vi "OAT Polar PG angle lines.vi"(6 "channel settings":T1 {"probe angle [deg]" max=360 step=1; "shaft rotating direction" items=["CCW", "CW"]}, 8 "grid measurements":T2 {"end angle" format="%.2f"; "start angle" format="%.2f"; "scale factors"."b" format="%.2f"; "scale factors"."a" format="%.2f"}, 9 "decade specs":cluster{"radius":i16, "label":string}[](array[cluster]), 11 "picture":picture) -> (3 "new picture":picture)   [LabVIEW 2017]
panel:
  in  "?":cluster{"angle":dbl, "min radius":i16}[](array[cluster])=[{"angle"=0.0, "min radius"=0}, {"angle"=15.0, "min radius"=25}, {"angle"=30.0, "min radius"=25}, {"angle"=45.0, "min radius"=10}, {"angle"=60.0, "min radius"=25}, {"angle"=75.0, "min radius"=25}] {"angle" format="%.2f"}
  # "To change the number of\nangle lines drawn add or\nremove elements from\nthis array.  (Changes\nwill only be temporary\nunless you make the new\nvalue the default and save\nthe VI.)\n\nAngle refers to the angle\nof the line in degrees.  The\nangles should be >=0 and\n<90, as these values are\nrepeated for each quadrant.\n\nMin radius refers to the\nsmallest size circle the\nlines should be drawn to."
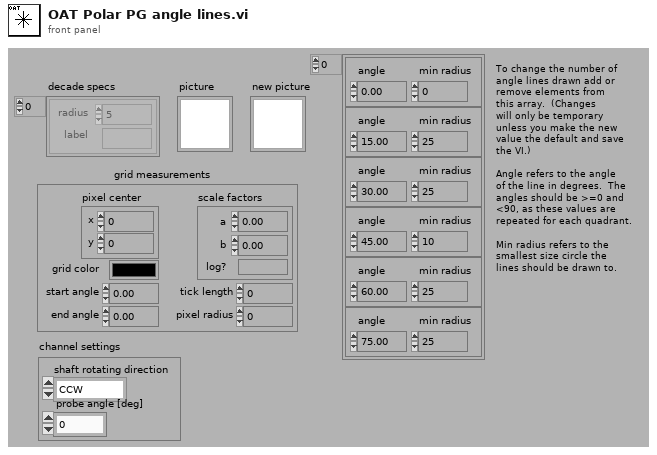
[diagram p1: front panel]
types:
  T1 = cluster{"shaft rotating direction":u16, "probe angle [deg]":u16}
  T2 = cluster{"pixel center":cluster{"x":i16, "y":i16}, "scale factors":cluster{"a":dbl, "b":dbl, "log?":bool}, "grid color":u32, "start angle":dbl, "end angle":dbl, "tick length":i16, "pixel radius":i32}
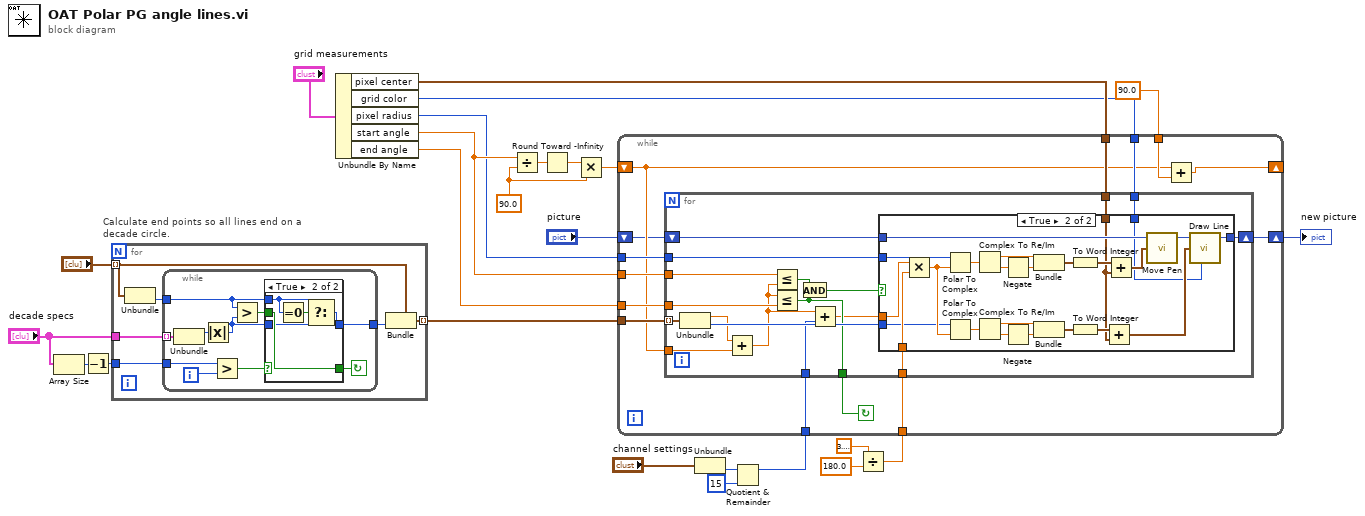
[diagram p0: block diagram]
diagram:
  w5 = 90.0
  n1 = Array Size(array="decade specs") -> (size(s)=w22:i32)
  n2 = Decrement(x=w22) -> (x-1=w20:i32)
  n3 = for "Calculate end points so all lines end on a decade circle." {
    tunnel: "?" -> [w28] mode=indexing
    tunnel: "decade specs" -> [w31]
    tunnel: w20 -> [w30]
    tunnel: [w26] -> w10 mode=indexing
    n4 = Unbundle(w28) -> ("min radius"=w29:i16)  [unwired: 1 out]
    n5 = while {
      tunnel: [w34] -> w27
      tunnel: w29 -> [w33]
      tunnel: w30 -> [w39]
      tunnel: w31 -> [w41] mode=indexing
      i -> [w40]
      stop <- w37 continue-if-true
      n6 = Unbundle(w41) -> ("radius"=w36:i16)  [unwired: 1 out]
      n7 = Absolute Value(x=w36) -> (abs(x)=w32:i16)
      n8 = Greater?(x=w39, y=w40) -> (0:w38:bool)
      n9 = Greater?(x=w33, y=w32) -> (0:w35:bool)
      n10 = case shown="True" w38 {
        selector: w38 -> [w43 _]
        tunnel: [w43 w48] -> w37
        tunnel: w32 -> [w42 w44]
        tunnel: w35 -> [_ w48]
        tunnel: [w42 w45] -> w34
        tunnel: w33 -> [_ w46]
        frame False {
          # "last element"
        }
        frame True {
          n11 = Equal To 0?(x=w46) -> (x = 0?=w47:bool)
          n12 = Select(t=w46, s=w47, f=w44) -> (s? t:f=w45:i16)
        }
      }
    }
    n13 = Bundle(cluster=w28, "min radius"=w27) -> (w26:cluster{"angle":dbl, "min radius":i16})  [unwired: 1 in]
  }
  n14 = Unbundle By Name("grid measurements") -> ("pixel center"=w24:cluster{"x":i16, "y":i16}, "grid color"=w9:u32, "pixel radius"=w11:i32, "start angle"=w13:dbl, "end angle"=w12:dbl)
  n15 = Divide(x=w13, y=w5) -> (x/y=w17:dbl)
  n16 = Round Toward -Infinity(1:w17) -> (0:w16:dbl)
  n17 = Multiply(x=w16, y=w5) -> (x*y=w15:dbl)
  n18 = Unbundle("channel settings") -> ("probe angle [deg]"=w3:u16)  [unwired: 1 out]
  n19 = Quotient & Remainder(x=w3, y=u16 15) -> (x-y*floor(x/y)=w1:u16)  [unwired: 1 out]
  n20 = Divide(x=3.141592653589793, y=180.0) -> (x/y=w14:dbl)
  n21 = while {
    shift-left: "picture" -> [w51]
    shift-right: [w50] -> w7
    tunnel: 90.0 -> [w54]
    tunnel: w9 -> [w55]
    tunnel: w24 -> [w56]
    tunnel: w10 -> [w57]
    tunnel: w11 -> [w58]
    tunnel: w12 -> [w59]
    tunnel: w13 -> [w60]
    tunnel: w14 -> [w61]
    shift-left: w15 -> [w53]
    shift-right: [w62] -> _
    tunnel: w1 -> [w49]
    stop <- w52 continue-if-true
    n22 = for {
      tunnel: w57 -> [w80] mode=indexing
      shift-right: [w78] -> w50
      shift-left: w51 -> [w79]
      tunnel: w56 -> [w77]
      tunnel: w55 -> [w76]
      tunnel: w61 -> [w75]
      tunnel: w60 -> [w71]
      tunnel: w59 -> [w70]
      tunnel: w58 -> [w69]
      tunnel: w53 -> [w68]
      tunnel: [w66] -> w52
      tunnel: w49 -> [w65]
      n23 = Unbundle(w80) -> ("angle"=w67:dbl, "min radius"=w74:i16)
      n24 = Add(x=w67, y=w68) -> (x+y=w64:dbl)
      n25 = Less Or Equal?(x=w71, y=w64) -> (x <= y?=w73:bool)
      n26 = Less Or Equal?(x=w64, y=w70) -> (x <= y?=w66:bool)
      n27 = And(x=w73, y=w66) -> (x .and. y?=w72:bool)
      n28 = Add(x=w64, y=w65) -> (x+y=w63:dbl)
      n29 = case shown="True" w72 {
        tunnel: w79 -> [w81 w91]
        tunnel: [w81 w90] -> w78
        tunnel: w77 -> [_ w89]
        tunnel: w76 -> [_ w88]
        tunnel: w69 -> [_ w87]
        tunnel: w75 -> [_ w86]
        tunnel: w74 -> [_ w85]
        tunnel: w63 -> [_ w84]
        frame False {
        }
        frame True {
          n30 = Multiply(x=w84, y=w86) -> (x*y=w98:dbl)
          n31 = Polar To Complex(1:w98, 2:w87) -> (0:w97:cdb)
          n32 = Polar To Complex(1:w98, 2:w85) -> (0:w94:cdb)
          n33 = Complex To Re/Im(x + iy=w97) -> (x=w99:dbl, y=w100:dbl)
          n34 = Complex To Re/Im(x + iy=w94) -> (x=w95:dbl, y=w96:dbl)
          n35 = Negate(x=w100) -> (-x=w82:dbl)
          n36 = Negate(x=w96) -> (-x=w83:dbl)
          n37 = Bundle(w99, w82) -> (w92:cluster{dbl, dbl})  [unwired: 1 in]
          n38 = Bundle(w95, w83) -> (w93:cluster{dbl, dbl})  [unwired: 1 in]
          n39 = To Word Integer(number=w92) -> (16bit integer=w102:cluster{i16, i16})
          n40 = To Word Integer(number=w93) -> (16bit integer=w101:cluster{i16, i16})
          n41 = Add(x=w101, y=w89) -> (x+y=w105:cluster{i16, i16})
          n42 = Add(x=w102, y=w89) -> (x+y=w104:cluster{i16, i16})
          n43 = call <vilib>:"Move Pen.vi"("new position"=w104, "picture"=w91) -> ("new picture"=w103:picture)  [unwired: 3 in]
          n44 = call <vilib>:"Draw Line.vi"("picture"=w103, "end point"=w105, "color(black)"=w88) -> ("new picture"=w90:picture)  [unwired: 6 in]
        }
      }
    }
    n45 = Add(x=w53, y=w54) -> (x+y=w62:dbl)
  }
  "new picture" <- w7
